vi "Reaffirm_ADAM_Outputs.vi"(3 "Reset Zeros as well":bool, 4 "Active Ch Indicies":i32[](array[numeric]), 5 "Channel Description":T1[](array[typedef]) {"Duty" format="%.0b"; "D" format="%#_5g"; "C" format="%#_5g"; "B" format="%#_5g"; "A" format="%#_5g"}, 6 "Current Channel Values":dbl[](array[numeric]) format="%.2f") -> (1 "Scan Comments":string[](array[string]))   [LabVIEW 2013]
uses:
  ADAM Client/Sub VIs/ADAM Controls/Ch_description_ADAM.ctl
  ADAM Client/Sub VIs/ADAM Controls/Module_type_ADAM.ctl
  ADAM Client/Sub VIs/ADAM Controls/Function_ADAM.ctl
  ADAM Client/Sub VIs/ADAM Controls/Channel_State.ctl
  ADAM Client/Sub VIs/ADAM Controls/Calib_type_ADAM.ctl
  ADAM Client/Sub VIs/ADAM Controls/Address.ctl
  ADAM_Global.vi
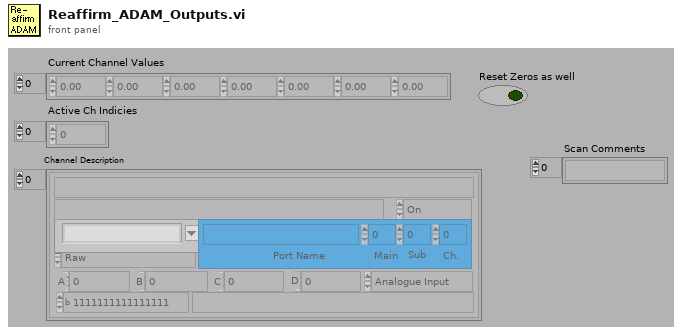
[diagram p1: front panel]
types:
  T1 = typedef "Ch_description_ADAM.ctl" = cluster{"Ch Name":string, "Type":T2, "Function":T3, "Ch State":T4, "Calibration type":T5, "A":dbl, "B":dbl, "C":dbl, "D":dbl, "Comments":string, "Address":T6, "String":string, "Duty":u16}
  T2 = typedef "Module_type_ADAM.ctl" = string
  T3 = typedef "Function_ADAM.ctl" = enum16{"Analogue Input", "Digital Input", "Event counter", "Event rate", "Analogue Output", "Digital Output", "Relay Output"}
  T4 = typedef "Channel_State.ctl" = enum16{"On", "Off", "Always On", "Always Off"}
  T5 = typedef "Calib_type_ADAM.ctl" = enum16{"Raw", "Bx + A", "Cx^2 + Bx + A", "Dx^3 + Cx^2 + Bx + A", "In Band", "Hi-Tec Q", "Hi-Tec M_dot", "Text"}
  T6 = typedef "Address.ctl" = cluster{"Main":i32, "Ch.":i32, "Sub":i32, "Port Name":string}
  T7 = typedef "Server_Control.ctl" = cluster{"Channel Name to control":string, "Channel sharing":enum16{"Channel Unshared", "Channel Shared by Rig", "Channel Shared by Group"}, "Default Value":dbl, "Client Array":string[], "Time Stamp":timestamp, "Do Not Reset":bool}
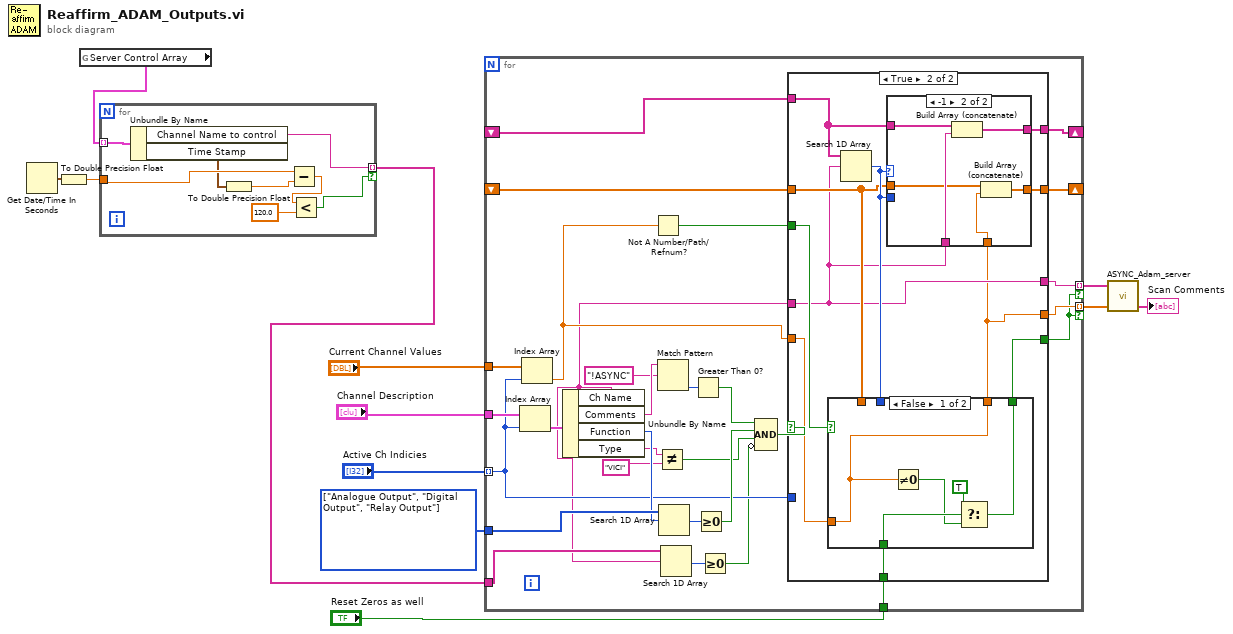
[diagram p0: block diagram]
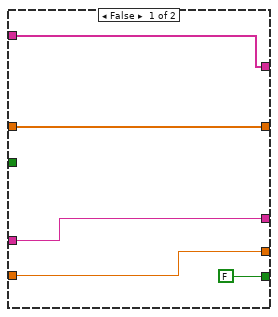
[diagram p2: hidden frame]
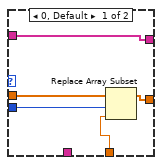
[diagram p3: hidden frame]
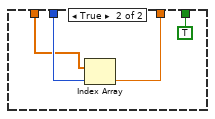
[diagram p4: hidden frame]
diagram:
  w10 = T3[] [enum."Analogue Output", enum."Digital Output", enum."Relay Output"] items=["Analogue Input", "Digital Input", "Event counter", "Event rate", "Analogue Output", "Digital Output", "Relay Output"]
  n1 = Get Date/Time In Seconds() -> (seconds since 1Jan1904=w6:timestamp)
  n2 = To Double Precision Float(number=w6) -> (double precision float=w5:dbl)
  n3 = global read "ADAM_Global.vi" "Server Control Array"() -> (w7:T7[])
  n4 = for {
    tunnel: w7 -> [w20] mode=indexing
    tunnel: w5 -> [w19]
    tunnel: [w14] -> w2 mode=indexing if=w13
    n5 = Unbundle By Name(w20) -> ("Channel Name to control"=w14:string, "Time Stamp"=w18:timestamp)
    n6 = To Double Precision Float(number=w18) -> (double precision float=w17:dbl)
    n7 = Subtract(x=w19, y=w17) -> (x-y=w16:dbl)
    n8 = Less?(x=w16, y=120.0) -> (x < y?=w13:bool)
  }
  n9 = for {
    tunnel: "Channel Description" -> [w40]
    tunnel: "Active Ch Indicies" -> [w38] mode=indexing
    tunnel: w10 -> [w49]
    tunnel: "Current Channel Values" -> [w39]
    shift-right: [w33] -> _
    shift-left: _ -> [w34]
    shift-right: [w31] -> _
    shift-left: _ -> [w32]
    tunnel: w2 -> [w28]
    tunnel: [w24] -> w4 mode=indexing if=w22
    tunnel: [w23] -> w3 mode=indexing if=w22
    tunnel: "Reset Zeros as well" -> [w21]
    n10 = Index Array(array=w40, index=w38) -> (element=w50:T1)
    n11 = Index Array(array=w39, index=w38) -> (element=w30:dbl)
    n12 = Unbundle By Name(w50) -> ("Ch Name"=w27:string, "Comments"=w47:string, "Function"=w48:T3, "Type"=w37:T2)
    n13 = Not A Number/Path/Refnum?(number/path/refnum=w30) -> (NaN/Path/Refnum?=w29:bool)
    n14 = Not Equal?(x=w37, y=T2 "VICI" ("Type")) -> (x != y?=w35:bool)
    n15 = Match Pattern(string=w47, regular expression="!ASYNC") -> (offset past match=w45:i32)  [unwired: 4 out]
    n16 = Search 1D Array(1D array=w49, element=w48) -> (index of element=w44:i32)  [unwired: 1 out]
    n17 = Search 1D Array(1D array=w28, element=w27) -> (index of element=w26:i32)  [unwired: 1 out]
    n18 = Greater Than 0?(x=w45) -> (x > 0?=w42:bool)
    n19 = Greater Or Equal To 0?(x=w44) -> (x >= 0?=w43:bool)
    n20 = Greater Or Equal To 0?(x=w26) -> (x >= 0?=w25:bool)
    n21 = Compound Arithmetic op=AND(w42, w43, w35, invert w25) -> (w41:bool)
    n22 = case shown="True" w41 {
      tunnel: w38 -> [_ _]
      tunnel: [w52 w58] -> w24
      tunnel: w27 -> [w53 w59]
      tunnel: [w53 w59] -> w23
      tunnel: w30 -> [w52 w63]
      tunnel: w34 -> [w55 w66]
      tunnel: [w55 w65] -> w33
      tunnel: w32 -> [w54 w61]
      tunnel: [w54 w64] -> w31
      tunnel: w29 -> [_ w60]
      tunnel: [FALSE w57] -> w22
      tunnel: w21 -> [_ w56]
      frame False {
      }
      frame True {
        n23 = Search 1D Array(1D array=w66, element=w59) -> (index of element=w62:i32)  [unwired: 1 out]
        n24 = case shown="False" w60 {
          tunnel: [w82 w84] -> w58
          tunnel: w63 -> [w82 _]
          tunnel: w62 -> [_ w86]
          tunnel: w61 -> [_ w85]
          tunnel: [w78 TRUE] -> w57
          tunnel: w56 -> [w81 _]
          frame False {
            n25 = Not Equal To 0?(x=w82) -> (x != 0?=w79:bool)
            n26 = Select(t=TRUE, s=w81, f=w79) -> (s? t:f=w78:bool)
          }
          frame True {
            n27 = Index Array(array=w85, index=w86) -> (element=w84:dbl)
          }
        }
        n28 = case shown="-1" w62 {
          tunnel: w66 -> [w71 w77]
          tunnel: w59 -> [_ w76]
          tunnel: [w71 w75] -> w65
          tunnel: w62 -> [w70 _]
          tunnel: w61 -> [w69 w74]
          tunnel: [w68 w72] -> w64
          tunnel: w58 -> [w67 w73]
          frame 0, Default {
            n29 = Replace Array Subset(array=w69, new element=w67, index=w70) -> (w68:dbl[])
          }
          frame -1 {
            n30 = Build Array (concatenate)(w77, w76) -> (w75:string[])
            n31 = Build Array (concatenate)(w74, w73) -> (w72:dbl[])
          }
        }
      }
    }
  }
  n32 = call "ASYNC_Adam_server.vi"("Values"=w4, "Channel Names"=w3) -> ("Scan Comments"=→"Scan Comments":string[])  [unwired: 1 in, 2 out]
